vi "List.vi"(8 "error in (no error)":errorcluster, 11 "LUnit Test Case V2 in":refnum<class "LUnit Test Case V2.lvclass">) -> (0 "error out":errorcluster, 2 "List of Runnables":string[](array[string]))   [LabVIEW 2020, in "LUnit Test Case V2.lvclass"]
uses:
  LUnit Test Case V2.lvclass
  LUnit Test Case V2.lvclass/LUnit Test Case V2.ctl
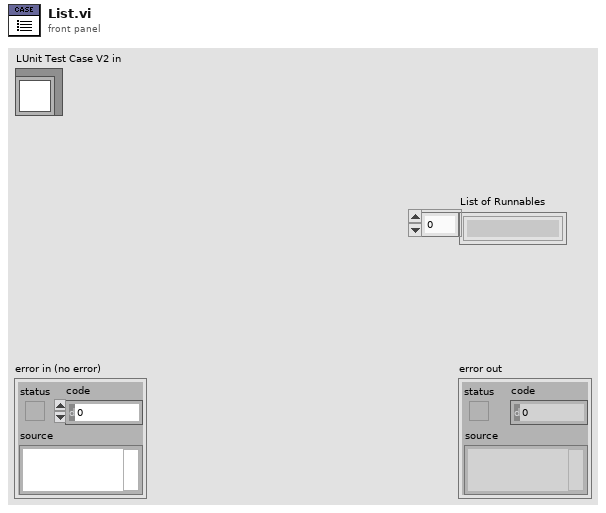
[diagram p1: front panel]
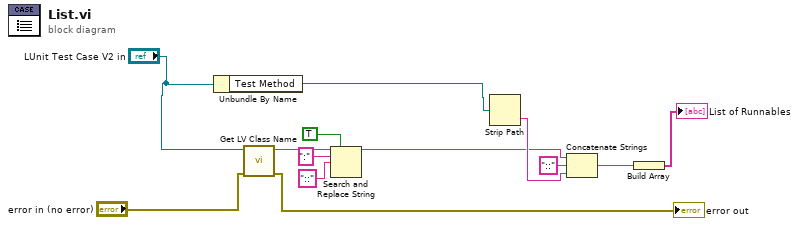
[diagram p0: block diagram]
diagram:
  n1 = Unbundle By Name("LUnit Test Case V2 in") -> ("Test Method"=w10:path)
  n2 = call <vilib>:"Get LV Class Name.vi"("error in (no error)"="error in (no error)", "object"="LUnit Test Case V2 in") -> ("error out"=→"error out":errorcluster, "class name"=w5:string)  [unwired: 8 in]
  n3 = Search and Replace String(replace all?=TRUE ("replace all? (F)"), input string=w5, search string=":", replace string="::" ("string")) -> (result string=w4:string)  [unwired: 4 in, 3 out]
  n4 = Strip Path(path=w10) -> (name=w8:string)  [unwired: 1 out]
  n5 = Concatenate Strings(w4, "::" ("string"), w8) -> (w7:string)
  n6 = Build Array(w7) -> (→"List of Runnables":string[])
